vi "pid.vi"(6 "dt [s]":dbl, 8 "error in (no error)":errorcluster, 9 "State":dbl, 10 "Reference":dbl, 11 "controller in":refnum<class "controller.lvclass">) -> (0 "error out":errorcluster, 2 "input":dbl, 3 "controller out":refnum<class "controller.lvclass">)   [LabVIEW 2025, in "controller.lvclass"]
uses:
  controller.lvclass
  controller.lvclass/controller.ctl
panel:
  in  "input minimum":dbl
  in  "input maximum":dbl=90.0
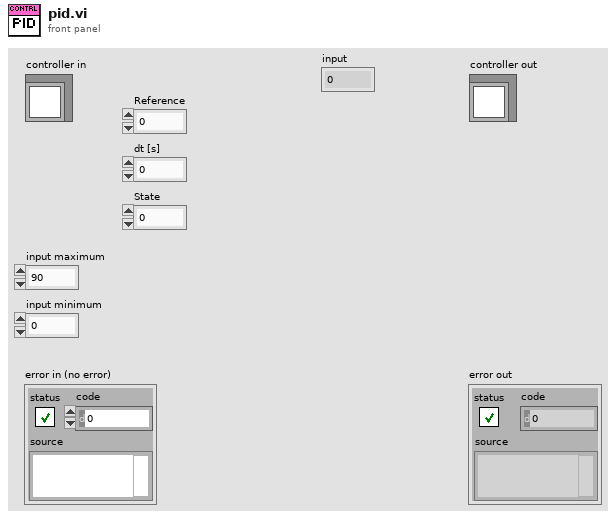
[diagram p1: front panel]
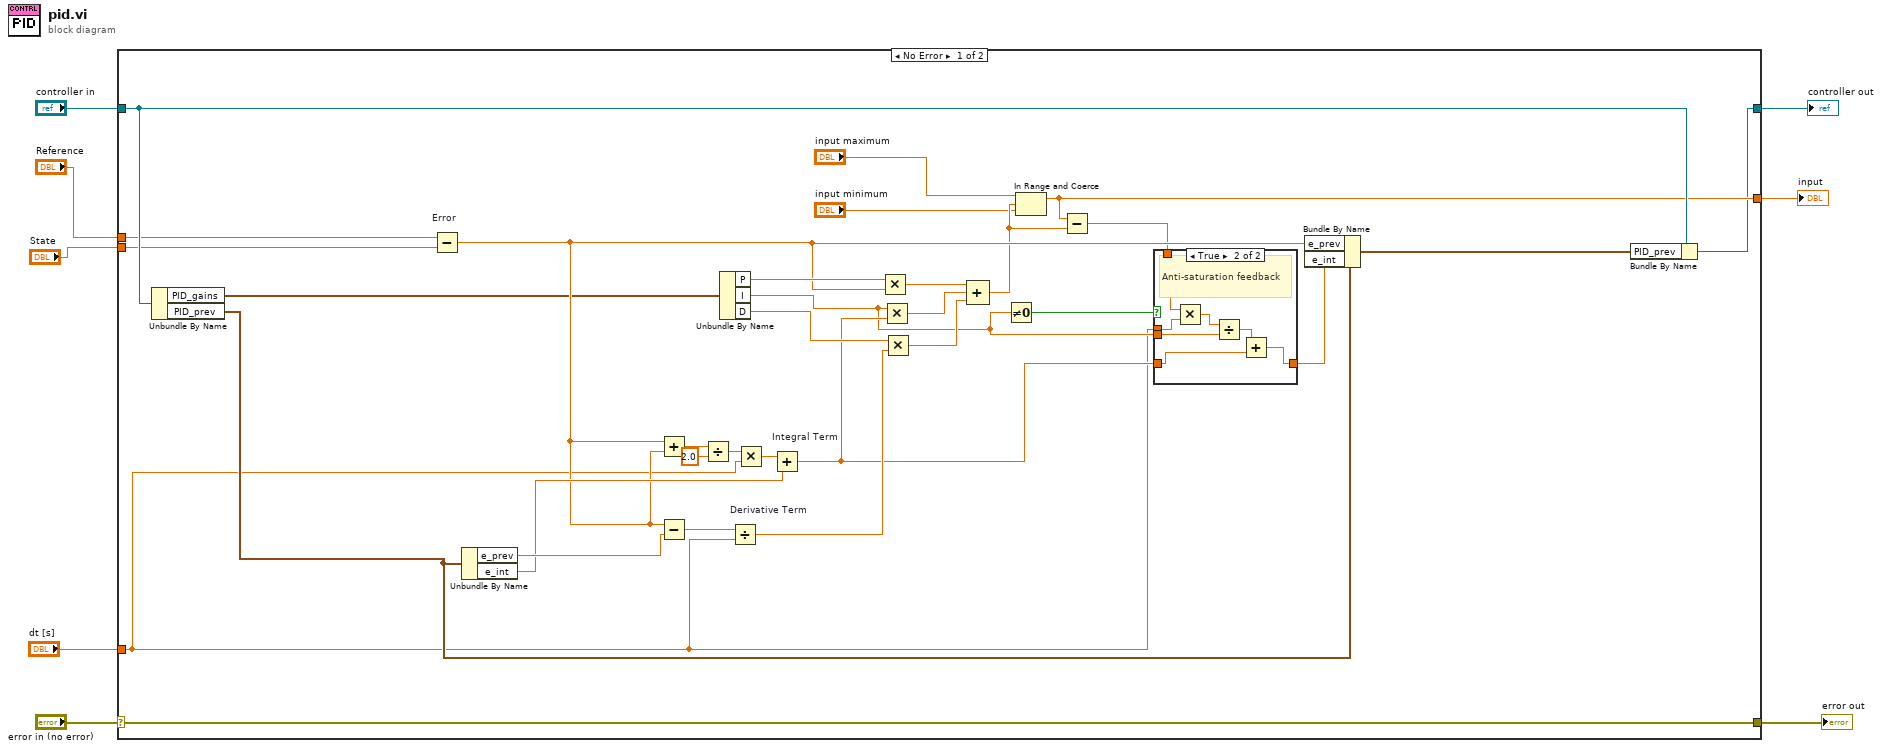
[diagram p0: block diagram]
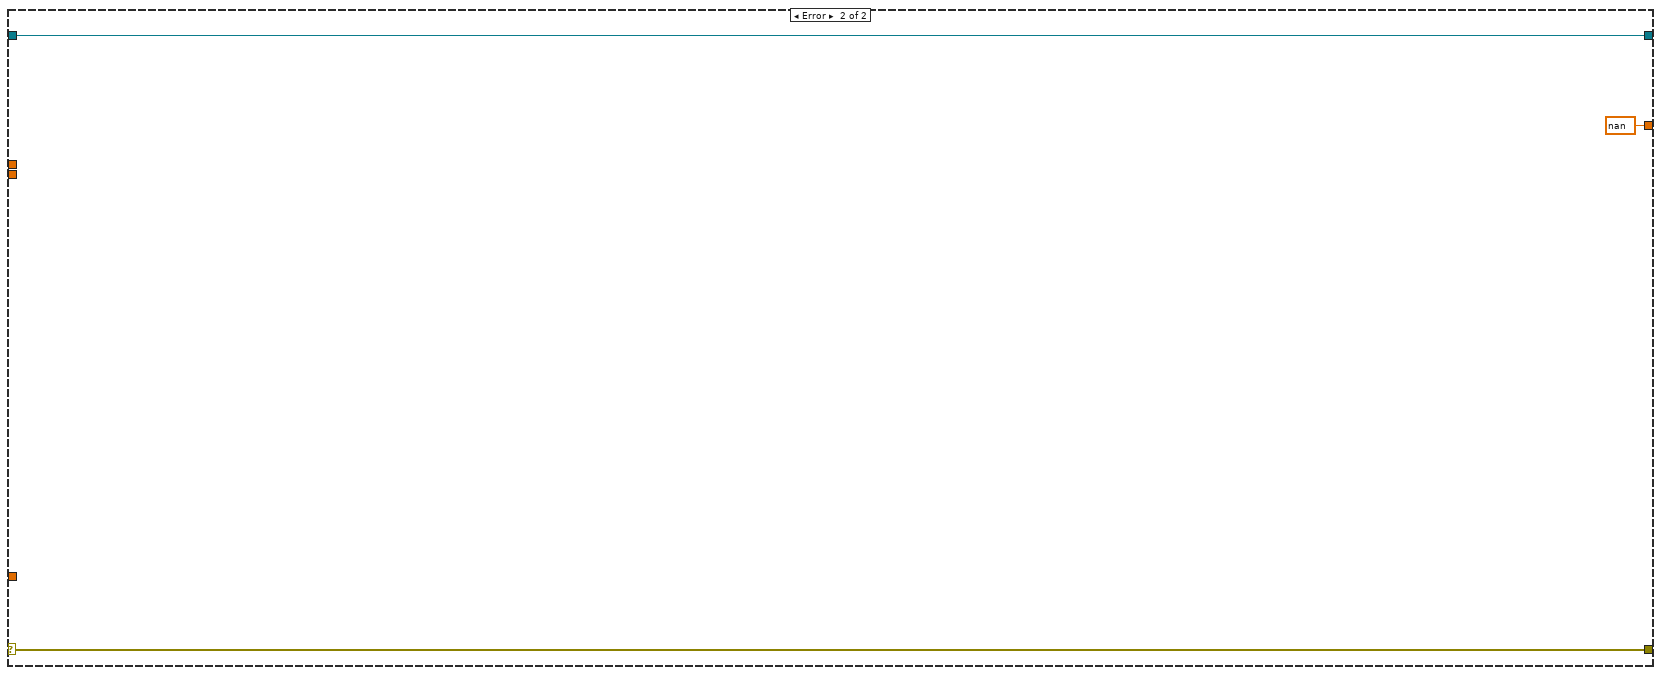
[diagram p3: hidden frame]
diagram:
  n1 = case shown="No Error" "error in (no error)" {
    selector: "error in (no error)" -> [w40 w51]
    tunnel: [w40 w51] -> w7
    tunnel: [w9 w50] -> w5
    tunnel: "controller in" -> [w17 w50]
    tunnel: "Reference" -> [w13 _]
    tunnel: "State" -> [w12 _]
    tunnel: "dt [s]" -> [w11 _]
    tunnel: [w10 nan ("input maximum")] -> w1
    frame No Error {
      n2 = Unbundle By Name(w17) -> ("PID_gains"=w18:cluster{"P":dbl, "I":dbl, "D":dbl}, "PID_prev"=w19:cluster{"e_prev":dbl, "e_int":dbl})
      n3 = Subtract "Error"(x=w13, y=w12) -> (x-y=w26:dbl)
      n4 = Unbundle By Name(w19) -> ("e_prev"=w34:dbl, "e_int"=w29:dbl)
      n5 = Add(x=w26, y=w26) -> (x+y=w31:dbl)
      n6 = Subtract(x=w26, y=w34) -> (x-y=w33:dbl)
      n7 = Divide(x=w31, y=2.0) -> (x/y=w28:dbl)
      n8 = Unbundle By Name(w18) -> ("P"=w39:dbl, "I"=w20:dbl, "D"=w38:dbl)
      n9 = Divide "Derivative Term"(x=w33, y=w11) -> (x/y=w32:dbl)
      n10 = Multiply(x=w28, y=w11) -> (x*y=w27:dbl)
      n11 = Add "Integral Term"(x=w27, y=w29) -> (x+y=w24:dbl)
      n12 = Multiply(x=w39, y=w26) -> (x*y=w37:dbl)
      n13 = Multiply(x=w20, y=w24) -> (x*y=w36:dbl)
      n14 = Multiply(x=w38, y=w32) -> (x*y=w35:dbl)
      n15 = Compound Arithmetic op=ADD(w37, w36, w35) -> (w22:dbl)
      n16 = Not Equal To 0?(x=w20) -> (x != 0?=w25:bool)
      n17 = In Range and Coerce(upper limit="input maximum", x=w22, lower limit="input minimum") -> (coerced(x)=w10:dbl)  [unwired: 1 out]
      n18 = Subtract(x=w10, y=w22) -> (x-y=w21:dbl)
      n19 = case shown="True" w25 {
        tunnel: w24 -> [w41 w43]
        tunnel: [w41 w42] -> w23
        tunnel: w21 -> [_ w48]
        tunnel: w11 -> [_ w47]
        tunnel: w20 -> [_ w45]
        frame False {
        }
        frame True {
          # "Anti-saturation feedback"
          n20 = Multiply(x=w48, y=w47) -> (x*y=w46:dbl)
          n21 = Divide(x=w46, y=w45) -> (x/y=w44:dbl)
          n22 = Add(x=w44, y=w43) -> (x+y=w42:dbl)
        }
      }
      n23 = Bundle By Name(cluster=w19, "e_prev"=w26, "e_int"=w23) -> (w16:cluster{"e_prev":dbl, "e_int":dbl})
      n24 = Bundle By Name(cluster=w17, "PID_prev"=w16) -> (w9:refnum<class "controller.lvclass">)
    }
    frame Error {
    }
  }
  "error out" <- w7
  "controller out" <- w5
  "input" <- w1
